vi "Square Root Mapping.vi"(0 "x":dbl, 2 "Min Distance":dbl, 3 "Max Distance":dbl, 5 "Angle":dbl) -> (7 "Angle to Turn":dbl)   [LabVIEW 2019]
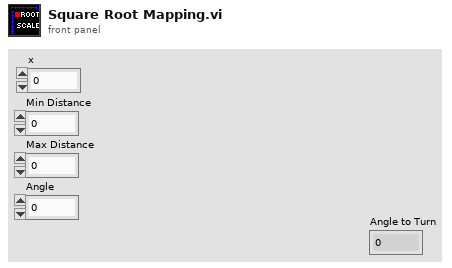
[diagram p1: front panel]
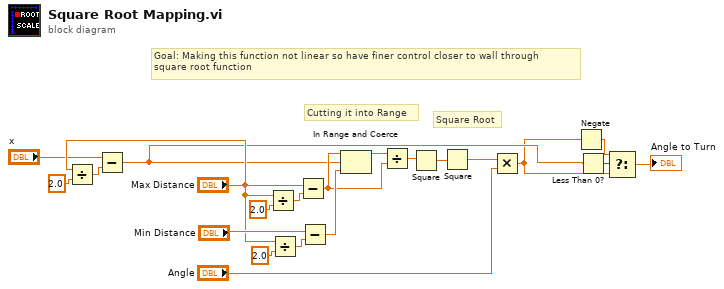
[diagram p0: block diagram]
diagram:
  # "Square Root"
  # "Goal: Making this function not linear so have finer control closer to wall through \nsquare root function"
  # "Cutting it into Range"
  n1 = Divide(x="Max Distance", y=2.0) -> (x/y=w19:dbl)
  n2 = Subtract(x="x", y=w19) -> (x-y=w4:dbl)
  n3 = Divide(x="Max Distance", y=2.0) -> (x/y=w16:dbl)
  n4 = Divide(x="Max Distance", y=2.0) -> (x/y=w15:dbl)
  n5 = Subtract(x="Max Distance", y=w16) -> (x-y=w11:dbl)
  n6 = Subtract(x="Min Distance", y=w15) -> (x-y=w12:dbl)
  n7 = In Range and Coerce(upper limit=w11, x=w4, lower limit=w12) -> (coerced(x)=w21:dbl)  [unwired: 1 out]
  n8 = Divide(x=w21, y=w11) -> (x/y=w9:dbl)
  n9 = Square(x=w9) -> (x^2=w8:dbl)
  n10 = Square(x=w8) -> (x^2=w7:dbl)
  n11 = Multiply(x=w7, y="Angle") -> (x*y=w3:dbl)
  n12 = Negate(x=w3) -> (-x=w2:dbl)
  n13 = Less Than 0?(x=w4) -> (x < 0?=w5:bool)
  n14 = Select(t=w2, s=w5, f=w3) -> (s? t:f=→"Angle to Turn":dbl)
